vi "usuario_contraseña.vi"(8 "error in":errorcluster) -> (0 "error out":errorcluster, 1 "Registro Flag":bool, 2 "Trabajador":string, 3 "Elemento a cola":string[](array[string]))   [LabVIEW 2017]
uses:
  <vilib>/NI/AMC/Update Message Routing Info.vi
  <vilib>/NI/AMC/Create Multiple Messages.vi
  <vilib>/NI/AMC/Read Termination Message.vi
  <vilib>/NI/AMC/Create Single Message.vi
  <vilib>/NI/AMC/Send Message.vi
  <vilib>/NI/AMC/Globals.vi
  Globals/Global.vi
  <vilib>/NI/AMC/AMC.lvlib
panel:
  in  "Cancel":bool
  in  "OK":bool
  in  "Cambiar contraseña":bool
  in  "Contraseña":string
  in  "Usuario":string
  # "INICIAR SESIÓN"
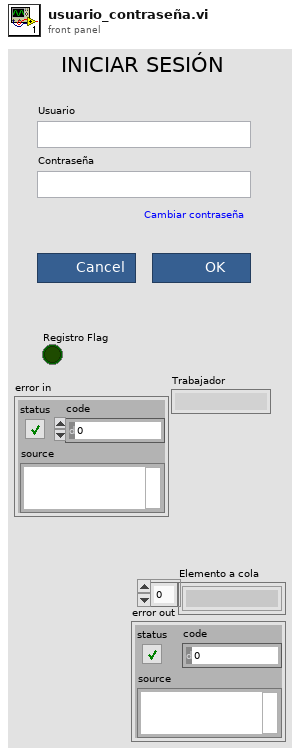
[diagram p1: front panel]
types:
  T1 = typedef "AMC.lvlib/Message Queue.ctl" = refnum<queue>
  T2 = cluster{"Nombre de usuario":string, "Contraseña":string, "Trabajador":string}[]
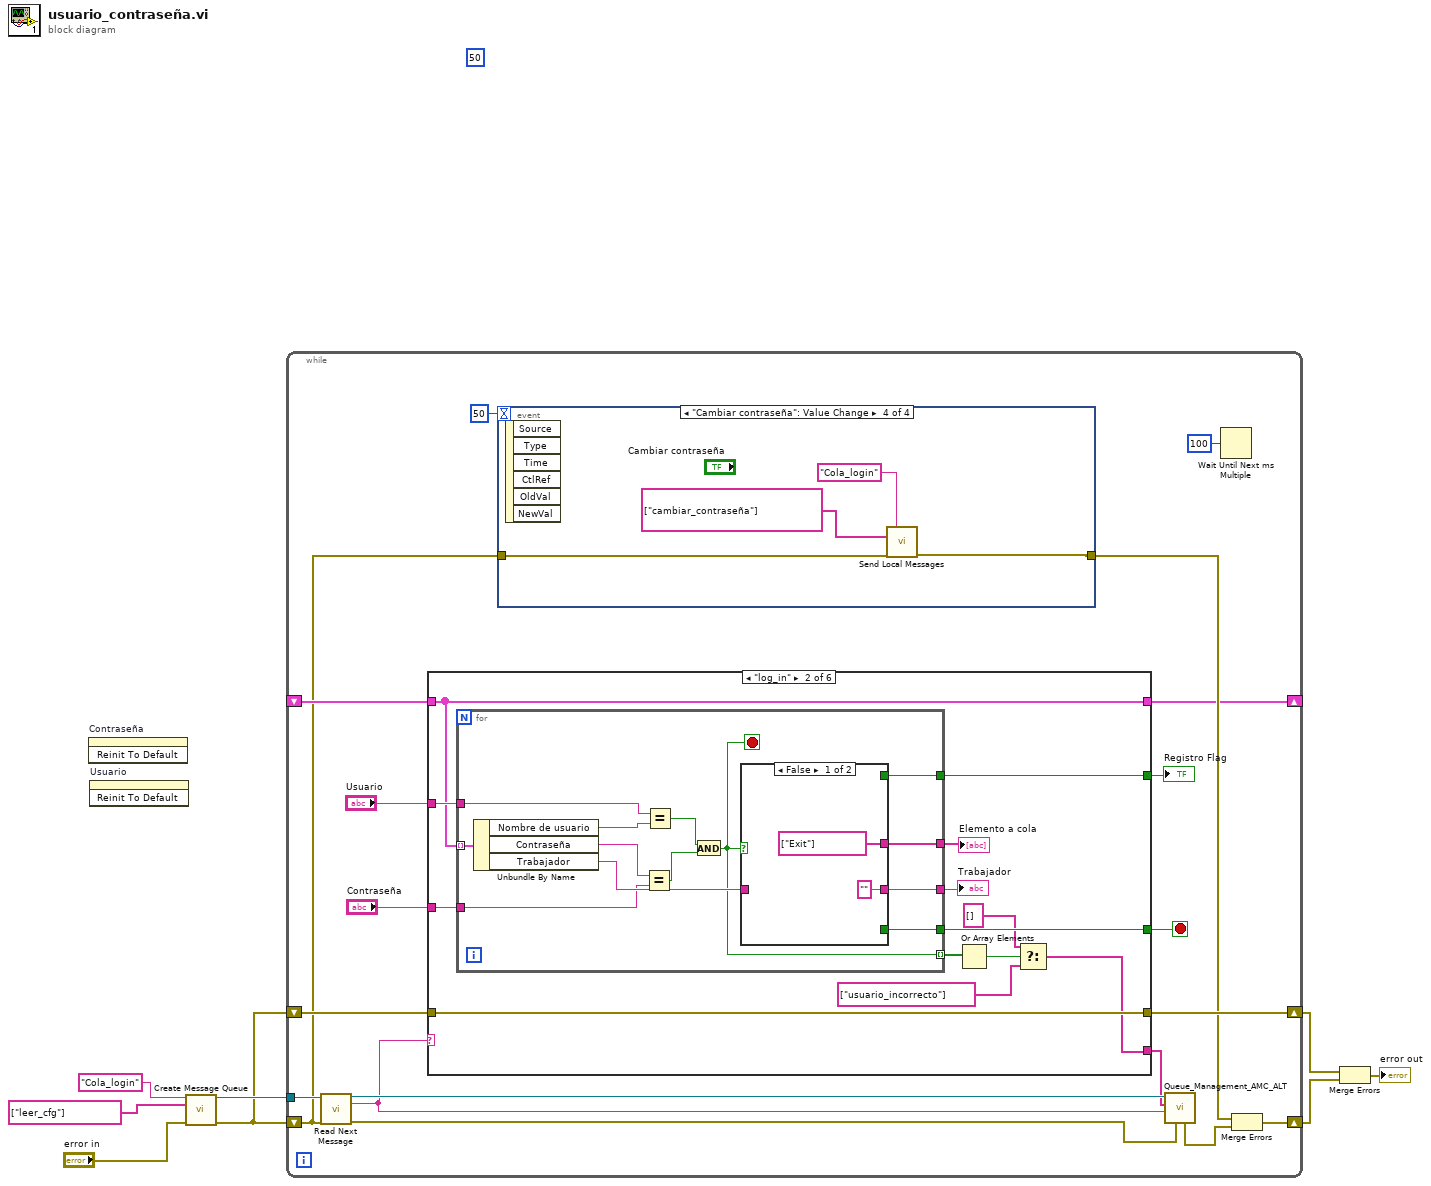
[diagram p0: block diagram]
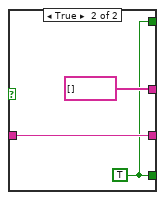
[diagram p3: hidden frame]
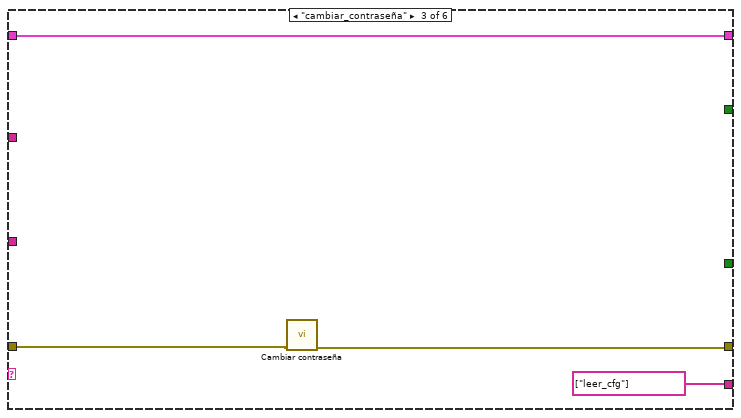
[diagram p4: hidden frame]
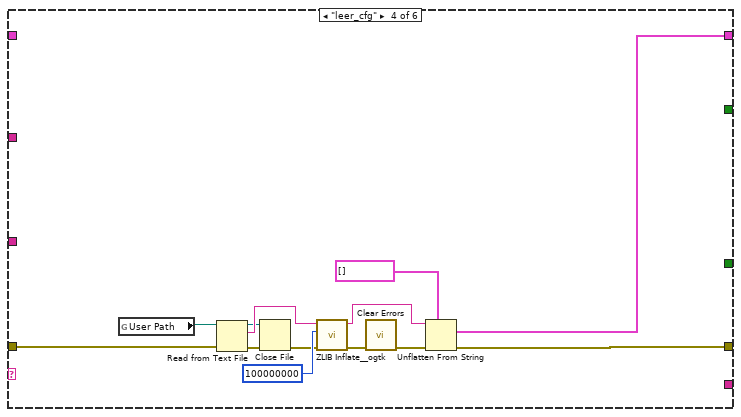
[diagram p5: hidden frame]
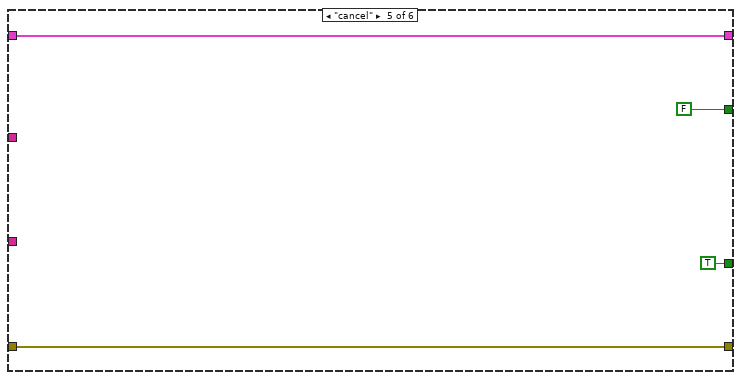
[diagram p6: hidden frame]
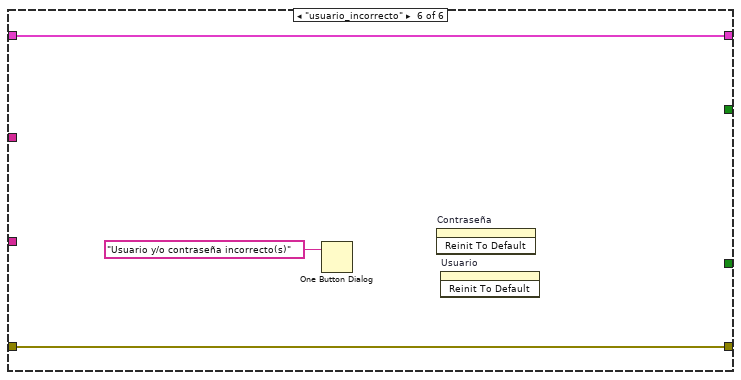
[diagram p7: hidden frame]
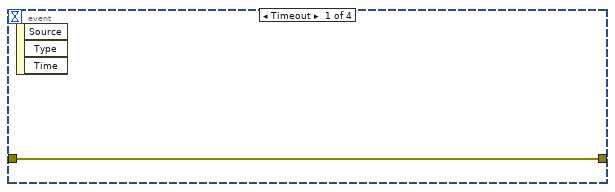
[diagram p8: hidden frame]
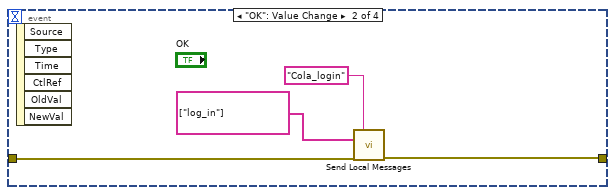
[diagram p9: hidden frame]
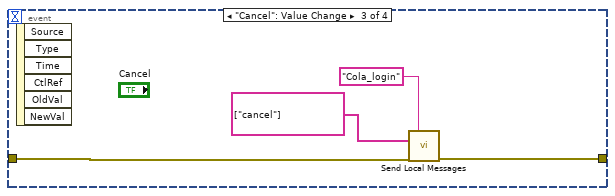
[diagram p10: hidden frame]
diagram:
  (unwired) 50
  n1 = invoke on="Contraseña" class="Str" method="Reinit To Default"() -> ()  [unwired: 3 in, 3 out]
  n2 = invoke on="Usuario" class="Str" method="Reinit To Default"() -> ()  [unwired: 3 in, 3 out]
  n3 = call <vilib>:"Create Message Queue.vi"("message queue name"="Cola_login", "initial message names"=string[] ["leer_cfg"], "error in"="error in") -> ("message queue out"=w7:T1, "error out"=w6:errorcluster)  [unwired: 11 in]
  n4 = while {
    tunnel: w7 -> [w23]
    shift-right: [w14] -> w4
    shift-left: w6 -> [w16]
    shift-right: [w17] -> w5
    shift-left: w6 -> [w18]
    shift-right: [w9] -> _
    shift-left: _ -> [w27]
    stop <- w24 stop-if-true
    n5 = call <vilib>:"Read Next Message.vi"("message queue in"=w23, "error in"=w16) -> ("message queue out"=w22:T1, "message name"=w21:string, "error out"=w19:errorcluster)  [unwired: 6 in, 5 out]
    n6 = case shown="\"log_in\"" w21 {
      tunnel: w27 -> [w28 w30 w61 _ w78 w82]
      tunnel: "Usuario" -> [_ w40 _ _ _ _]
      tunnel: "Contraseña" -> [_ w39 _ _ _ _]
      tunnel: [_ w38 _ _ TRUE _] -> w24
      tunnel: [_ w32 string[] ["leer_cfg"] ("initial message names") _ _ _] -> w20
      tunnel: w18 -> [w29 w37 w64 w75 w81 w83]
      tunnel: [w29 w37 w63 w74 w81 w83] -> w17
      tunnel: [_ w31 _ _ FALSE _] -> w12
      tunnel: [w28 w30 w61 w73 w78 w82] -> w9
      frame "False", Default {
      }
      frame "log_in" {
        n7 = for {
          tunnel: w30 -> [w55] mode=indexing
          tunnel: [w49] -> w42
          tunnel: [w48] -> w41
          tunnel: w40 -> [w47]
          tunnel: w39 -> [w46]
          tunnel: [w45] -> w38
          tunnel: [w44] -> w36 mode=indexing
          tunnel: [w43] -> w31
          stop <- w44 stop-if-true
          n8 = Unbundle By Name(w55) -> ("Nombre de usuario"=w54:string, "Contraseña"=w53:string, "Trabajador"=w50:string)
          n9 = Equal?(x=w53, y=w46) -> (x = y?=w51:bool)
          n10 = Equal?(x=w47, y=w54) -> (x = y?=w52:bool)
          n11 = And(x=w52, y=w51) -> (x .and. y?=w44:bool)
          n12 = case shown="False" w44 {
            tunnel: w50 -> [_ w60]
            tunnel: ["" ("Trabajador") w60] -> w49
            tunnel: [string[] ["Exit"] ("Trabajador") string[] [] ("Trabajador")] -> w48
            tunnel: [_ w58] -> w45
            tunnel: [_ w58] -> w43
            frame False {
            }
            frame True {
              w58 = TRUE
            }
          }
        }
        "Trabajador" <- w42
        "Elemento a cola" <- w41
        n13 = Or Array Elements(Boolean array=w36) -> (logical OR=w35:bool)
        n14 = Select(t=string[] [] ("Elementos a cola"), s=w35, f=string[] ["usuario_incorrecto"]) -> (s? t:f=w32:string[])
      }
      frame "cambiar_contraseña" {
        n15 = call "Cambiar contraseña.vi"("error in"=w64) -> ("error out"=w63:errorcluster)  [unwired: 10 in]
      }
      frame "leer_cfg" {
        n16 = global read "Global.vi" "User Path"() -> (w77:path)
        n17 = Read from Text File(file (use dialog)=w77, error in=w75) -> (refnum out=w67:refnum<file>, text=w76:string, error out=w66:errorcluster)  [unwired: 2 in, 1 out]
        n18 = Close File(refnum=w67, error in=w66) -> (error out=w65:errorcluster)  [unwired: 1 out]
        n19 = call <userlib>:"ZLIB Inflate__ogtk.vi"("error in (no error)"=w65, "expected length (try out)"=100000000, "input"=w76) -> ("error out"=w71:errorcluster, "inflated output"=w68:string)  [unwired: 2 in, 1 out]
        n20 = call <vilib>:"Clear Errors.vi"("error in (no error)"=w71) -> ("error out"=w70:errorcluster)  [unwired: 5 in, 1 out]
        n21 = Unflatten From String(type=T2 [] ("Array"), binary string=w68, error in (no error)=w70) -> (value=w73:T2, error out=w74:errorcluster)  [unwired: 2 in, 1 out]
      }
      frame "cancel" {
      }
      frame "usuario_incorrecto" {
        n22 = One Button Dialog(message="Usuario y/o contraseña incorrecto(s)") -> ()  [unwired: 1 in, 1 out]
        n23 = invoke on="Contraseña" class="Str" method="Reinit To Default"() -> ()  [unwired: 3 in, 3 out]
        n24 = invoke on="Usuario" class="Str" method="Reinit To Default"() -> ()  [unwired: 3 in, 3 out]
      }
    }
    "Registro Flag" <- w12
    n25 = event shown="[3] \"Cambiar contraseña\": Value Change" {
      selector: _ -> [_ _ _ _]
      dyn-events: _ -> [_ _ _ _]
      timeout: 50 -> [_ _ _ _]
      tunnel: w16 -> [w85 w86 w92 w95]
      tunnel: [w85 w87 w91 w94] -> w13
      event Timeout {
        n26 = event-data() -> ()  [unwired: 1 in, 3 out]
      }
      event "OK": Value Change {
        n27 = event-data() -> ()  [unwired: 1 in, 6 out]
        n28 = call <vilib>:"Send Local Messages.vi"("receiver process (\"\" - local)"="Cola_login" ("receiver process (\"\" - local)"), "message names"=string[] ["log_in"] ("message name"), "error in"=w86) -> ("error out"=w87:errorcluster)  [unwired: 10 in, 2 out]
      }
      event "Cancel": Value Change {
        n29 = event-data() -> ()  [unwired: 1 in, 6 out]
        n30 = call <vilib>:"Send Local Messages.vi"("receiver process (\"\" - local)"="Cola_login" ("receiver process (\"\" - local)"), "message names"=string[] ["cancel"] ("message name"), "error in"=w92) -> ("error out"=w91:errorcluster)  [unwired: 10 in, 2 out]
      }
      event "Cambiar contraseña": Value Change {
        n31 = event-data() -> ()  [unwired: 1 in, 6 out]
        n32 = call <vilib>:"Send Local Messages.vi"("receiver process (\"\" - local)"="Cola_login" ("receiver process (\"\" - local)"), "message names"=string[] ["cambiar_contraseña"] ("message name"), "error in"=w95) -> ("error out"=w94:errorcluster)  [unwired: 10 in, 2 out]
      }
    }
    n33 = call "Queue_Management_AMC_ALT.vi"("queue error in"=w19, "Case"=w21, "Elementos a cola"=w20, "message queue in"=w22) -> ("queue error out"=w15:errorcluster)  [unwired: 4 in, 3 out]
    n34 = Wait Until Next ms Multiple(millisecond multiple=u32 100) -> ()  [unwired: 1 out]
    n35 = Merge Errors(w13, w15) -> (w14:errorcluster)
  }
  n36 = Merge Errors(w5, w4) -> (→"error out":errorcluster)
